vi "Bank Tester.vi"(8 "错误输入":cluster{"状态":bool, "代码":i32, "源":string}) -> (0 "错误输出":cluster{"状态":bool, "代码":i32, "源":string})   [LabVIEW 2012]
uses:
  Account Info.ctl
  Stop.vi
panel:
  in  "命令":T1
  in  "存款额":dbl
  in  "取款额":dbl
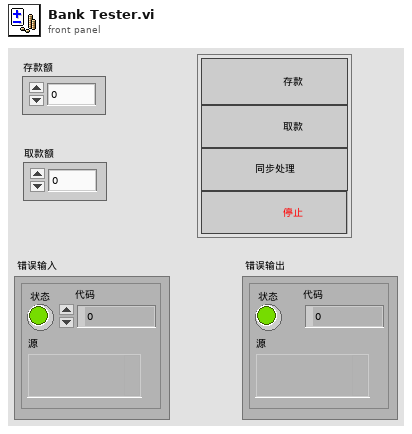
[diagram p1: front panel]
types:
  T1 = cluster{"存款":bool, "取款":bool, "同步":bool, "并发2":bool}
  T2 = typedef "Account Info.ctl" = cluster{"银行集合点":T3, "取款队列":refnum<queue>, "存款队列":refnum<queue>}
  T3 = typedef "Rendezvous RefNum" = refnum<k1>
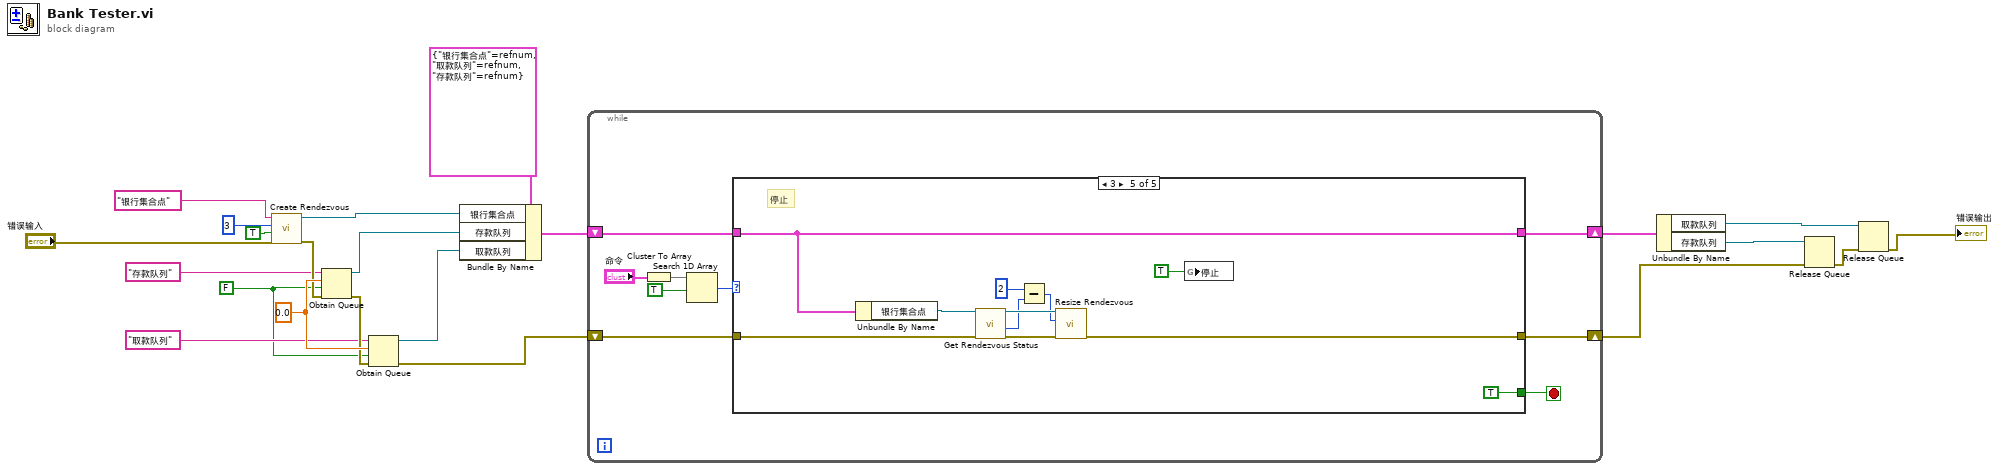
[diagram p0: block diagram]
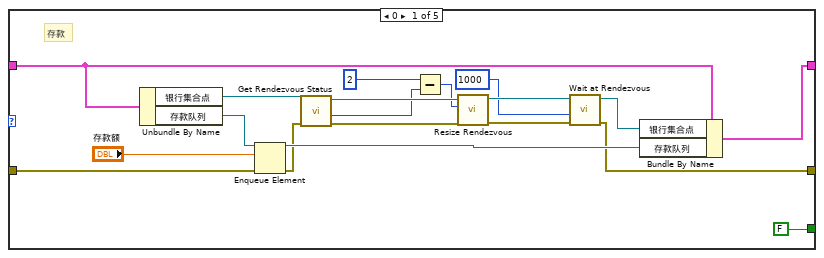
[diagram p2: hidden frame]
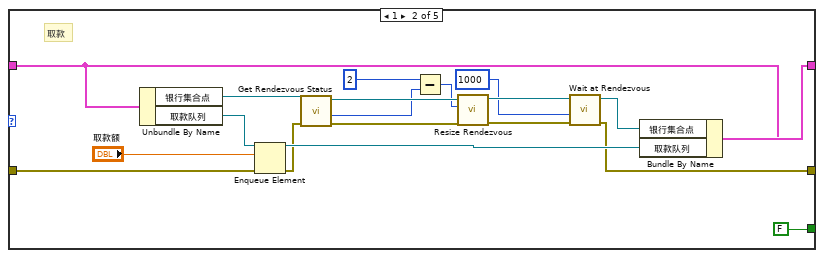
[diagram p3: hidden frame]
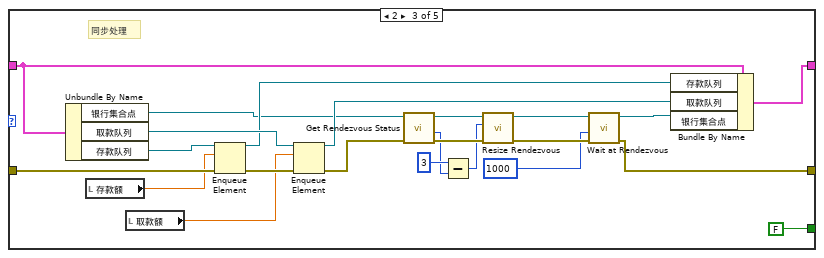
[diagram p4: hidden frame]
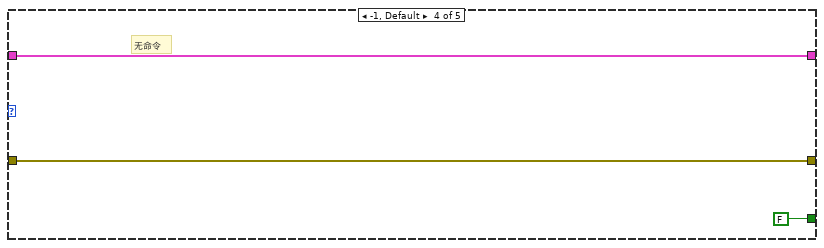
[diagram p5: hidden frame]
diagram:
  w1 = FALSE ("返回现有(F)")
  w21 = 0.0
  n1 = call <vilib>:"Create Rendezvous.vi"("error in (no error)"="错误输入", "return existing (F)"=TRUE ("返回现有(F)"), "size (2)"=3 ("大小(2)"), "name (unnamed)"="银行集合点" ("名称（未命名）")) -> ("error out"=w20:errorcluster, "rendezvous"=w22:T3)  [unwired: 1 in, 1 out]
  n2 = Obtain Queue ("获取队列引用")(name (unnamed)="存款队列" ("名称（未命名）"), element data type=w21, create if not found? (T)=w1, error in (no error)=w20) -> (queue out=w18:refnum<queue>, error out=w19:errorcluster)  [unwired: 1 in, 1 out]
  n3 = Obtain Queue ("获取队列引用")(name (unnamed)="取款队列" ("名称（未命名）"), element data type=w21, create if not found? (T)=w1, error in (no error)=w19) -> (queue out=w17:refnum<queue>, error out=w9:errorcluster)  [unwired: 1 in, 1 out]
  n4 = Bundle By Name ("按名称捆绑")(cluster=T2 {"银行集合点"=refnum, "取款队列"=refnum, "存款队列"=refnum} ("帐户信息"), "银行集合点"=w22, "存款队列"=w18, "取款队列"=w17) -> (w11:T2)
  n5 = while {
    shift-right: [w25] -> w4
    shift-left: w9 -> [w24]
    shift-right: [w26] -> w8
    shift-left: w11 -> [w28]
    stop <- w23 stop-if-true
    n6 = Cluster To Array ("簇至数组转换")(cluster="命令") -> (array=w30:bool[])
    n7 = Search 1D Array ("搜索一维数组")(1D array=w30, element=TRUE ("元素")) -> (index of element=w29:i32)  [unwired: 1 in]
    n8 = case shown="3" w29 {
      tunnel: w28 -> [w42 w62 w88 w95 w104]
      tunnel: w24 -> [w48 w68 w85 w94 w100]
      tunnel: [w43 w63 w89 w95 w104] -> w26
      tunnel: [w41 w61 w87 w94 w96] -> w25
      tunnel: [FALSE FALSE FALSE FALSE TRUE] -> w23
      frame 0 {
        # "存款"
        n9 = Unbundle By Name ("按名称解除捆绑")(w42) -> ("银行集合点"=w36:T3, "存款队列"=w50:refnum<queue>)
        n10 = Enqueue Element ("元素入队列")(queue=w50, element="存款额", error in (no error)=w48) -> (queue out=w44:refnum<queue>, error out=w38:errorcluster)  [unwired: 1 in, 1 out]
        n11 = call <vilib>:"Get Rendezvous Status.vi"("error in (no error)"=w38, "rendezvous"=w36) -> ("error out"=w37:errorcluster, "size"=w33:i32, "rendezvous out"=w35:T3)  [unwired: 5 in, 2 out]
        n12 = Subtract ("减")(x=2 ("大小变化(0)"), y=w33) -> (x-y=w32:i32)
        n13 = call <vilib>:"Resize Rendezvous.vi"("error in (no error)"=w37, "size change (0)"=w32, "rendezvous"=w35) -> ("error out"=w47:errorcluster, "rendezvous out"=w46:T3)  [unwired: 2 in, 1 out]
        n14 = call <vilib>:"Wait at Rendezvous.vi"("error in (no error)"=w47, "ms timeout (-1)"=1000 ("毫秒超时(-1)"), "rendezvous"=w46) -> ("error out"=w41:errorcluster, "rendezvous out"=w45:T3)  [unwired: 2 in, 1 out]
        n15 = Bundle By Name ("按名称捆绑")(cluster=w42, "银行集合点"=w45, "存款队列"=w44) -> (w43:T2)
      }
      frame 1 {
        # "取款"
        n16 = Unbundle By Name ("按名称解除捆绑")(w62) -> ("银行集合点"=w56:T3, "取款队列"=w69:refnum<queue>)
        n17 = Enqueue Element ("元素入队列")(queue=w69, element="取款额", error in (no error)=w68) -> (queue out=w64:refnum<queue>, error out=w58:errorcluster)  [unwired: 1 in, 1 out]
        n18 = call <vilib>:"Get Rendezvous Status.vi"("error in (no error)"=w58, "rendezvous"=w56) -> ("error out"=w57:errorcluster, "size"=w53:i32, "rendezvous out"=w55:T3)  [unwired: 5 in, 2 out]
        n19 = Subtract ("减")(x=2 ("大小变化(0)"), y=w53) -> (x-y=w52:i32)
        n20 = call <vilib>:"Resize Rendezvous.vi"("error in (no error)"=w57, "size change (0)"=w52, "rendezvous"=w55) -> ("error out"=w67:errorcluster, "rendezvous out"=w66:T3)  [unwired: 2 in, 1 out]
        n21 = call <vilib>:"Wait at Rendezvous.vi"("error in (no error)"=w67, "ms timeout (-1)"=1000 ("毫秒超时(-1)"), "rendezvous"=w66) -> ("error out"=w61:errorcluster, "rendezvous out"=w65:T3)  [unwired: 2 in, 1 out]
        n22 = Bundle By Name ("按名称捆绑")(cluster=w62, "银行集合点"=w65, "取款队列"=w64) -> (w63:T2)
      }
      frame 2 {
        # "同步处理"
        n23 = Unbundle By Name ("按名称解除捆绑")(w88) -> ("银行集合点"=w76:T3, "取款队列"=w92:refnum<queue>, "存款队列"=w86:refnum<queue>)
        n24 = local read "存款额"() -> (w80:dbl)
        n25 = local read "取款额"() -> (w79:dbl)
        n26 = Enqueue Element ("元素入队列")(queue=w86, element=w80, error in (no error)=w85) -> (queue out=w83:refnum<queue>, error out=w84:errorcluster)  [unwired: 1 in, 1 out]
        n27 = Enqueue Element ("元素入队列")(queue=w92, element=w79, error in (no error)=w84) -> (queue out=w81:refnum<queue>, error out=w75:errorcluster)  [unwired: 1 in, 1 out]
        n28 = call <vilib>:"Get Rendezvous Status.vi"("error in (no error)"=w75, "rendezvous"=w76) -> ("error out"=w74:errorcluster, "size"=w71:i32, "rendezvous out"=w73:T3)  [unwired: 5 in, 2 out]
        n29 = Subtract ("减")(x=3 ("大小变化(0)"), y=w71) -> (x-y=w70:i32)
        n30 = call <vilib>:"Resize Rendezvous.vi"("error in (no error)"=w74, "size change (0)"=w70, "rendezvous"=w73) -> ("error out"=w91:errorcluster, "rendezvous out"=w90:T3)  [unwired: 2 in, 1 out]
        n31 = call <vilib>:"Wait at Rendezvous.vi"("error in (no error)"=w91, "ms timeout (-1)"=1000 ("毫秒超时(-1)"), "rendezvous"=w90) -> ("error out"=w87:errorcluster, "rendezvous out"=w82:T3)  [unwired: 2 in, 1 out]
        n32 = Bundle By Name ("按名称捆绑")(cluster=w88, "存款队列"=w83, "取款队列"=w81, "银行集合点"=w82) -> (w89:T2)
      }
      frame -1, Default {
        # "无命令"
      }
      frame 3 {
        # "停止"
        n33 = Unbundle By Name ("按名称解除捆绑")(w104) -> ("银行集合点"=w101:T3)
        n34 = call <vilib>:"Get Rendezvous Status.vi"("error in (no error)"=w100, "rendezvous"=w101) -> ("error out"=w103:errorcluster, "size"=w99:i32, "rendezvous out"=w102:T3)  [unwired: 5 in, 2 out]
        n35 = Subtract ("减")(x=2, y=w99) -> (x-y=w97:i32)
        n36 = call <vilib>:"Resize Rendezvous.vi"("error in (no error)"=w103, "size change (0)"=w97, "rendezvous"=w102) -> ("error out"=w96:errorcluster)  [unwired: 2 in, 2 out]
        n37 = global write "Stop.vi" "停止"(TRUE ("停止")) -> ()
      }
    }
  }
  n38 = Unbundle By Name ("按名称解除捆绑")(w8) -> ("取款队列"=w6:refnum<queue>, "存款队列"=w7:refnum<queue>)
  n39 = Release Queue ("释放队列引用")(queue=w7, error in (no error)=w4) -> (error out=w5:errorcluster)  [unwired: 1 in, 2 out]
  n40 = Release Queue ("释放队列引用")(queue=w6, error in (no error)=w5) -> (error out=→"错误输出":errorcluster)  [unwired: 1 in, 2 out]
